vi "Exit.vi"(8 "error in (no error)":errorcluster, 11 "Init In":refnum<class "Init.lvclass">) -> (0 "error out":errorcluster, 3 "Init Out":refnum<class "Init.lvclass">)   [LabVIEW 2024, in "Test States.lvlib" / "Init.lvclass"]
doc: "This is an abstract method. Override this method to define the behavior when you leave the state."
uses:
  Init.lvclass
  C:/Program Files/National Instruments/LabVIEW 2024/vi.lib/ActorFramework/Actor/Actor.lvclass
  <vilib>/ActorFramework/Actor/Actor.lvclass/Actor.ctl
  Test UI Messages/Update Log Msg/Update Log Msg.lvclass/Update Log Msg.ctl
  <vilib>/ActorFramework/Message Enqueuer/Message Enqueuer.lvclass/Message Enqueuer.ctl
  <vilib>/ActorFramework/Message Enqueuer/Enqueue.vi
  Test UI Messages/Update Log Msg/Update Log Msg.lvclass
  C:/Program Files/National Instruments/LabVIEW 2024/vi.lib/ActorFramework/Message/Message.lvclass
  <vilib>/ActorFramework/Message Priority Queue/Priority Enqueue.vi
  Test State/Test State.lvclass
  <vilib>/ActorFramework/Actor/Actor.lvclass
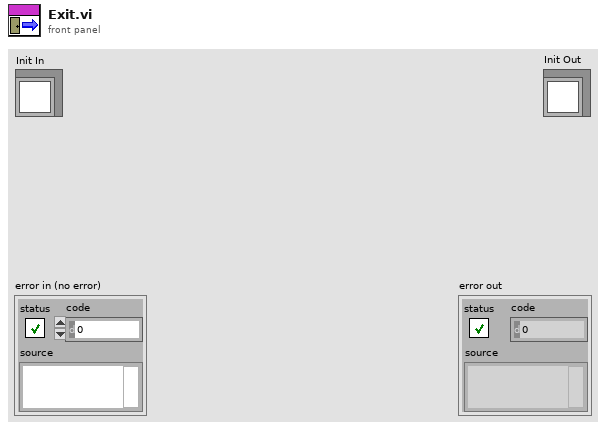
[diagram p1: front panel]
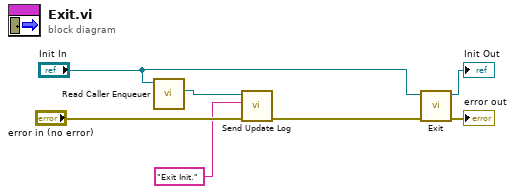
[diagram p0: block diagram]
diagram:
  n1 = call <vilib>:"Read Caller Enqueuer.vi"("Actor"="Init In") -> ("Caller Enqueuer"=w4:refnum<class "Message Enqueuer.lvclass">)  [unwired: 10 in]
  n2 = call "Send Update Log.vi"("error in (no error)"="error in (no error)", "Message"="Exit Init.", "Message Enqueuer"=w4) -> ("error out"=w2:errorcluster)  [unwired: 7 in, 1 out]
  n3 = call-parent "Exit.vi"("error in (no error)"=w2, "Old State"="Init In") -> ("error out"=→"error out":errorcluster, "New State"=→"Init Out":refnum<class "Init.lvclass">)  [unwired: 8 in]
